vi "find object distance in direction.vi"(9 "direction":dbl, 10 "point":cluster{"x":i16, "y":i16}, 11 "raster image":bool[][](array[boolean])) -> (2 "distance":sgl)   [LabVIEW 2009]
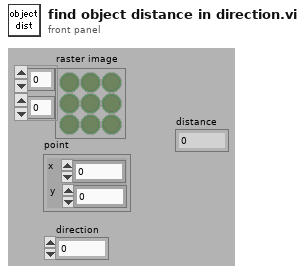
[diagram p1: front panel]
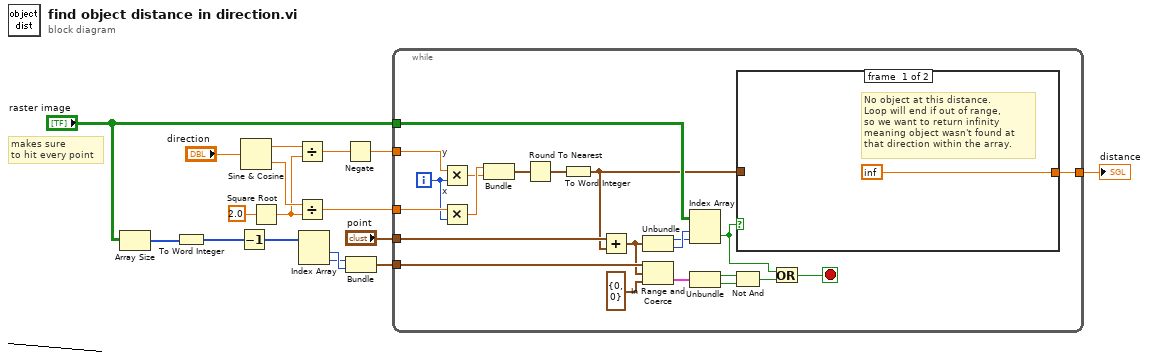
[diagram p0: block diagram]
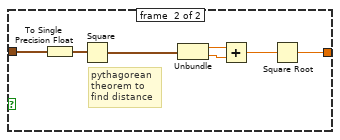
[diagram p2: hidden frame]
diagram:
  # "makes sure\nto hit every point"
  n1 = Array Size(array="raster image") -> (size(s)=w7:i32[])
  n2 = To Word Integer(number=w7) -> (16bit integer=w5:i16[])
  n3 = Decrement(x=w5) -> (x-1=w6:i16[])
  n4 = Sine & Cosine(0:"direction") -> (1:w14:dbl, 2:w15:dbl)
  n5 = Square Root(x=2.0) -> (sqrt(x)=w13:dbl)
  n6 = Divide(x=w14, y=w13) -> (x/y=w12:dbl)
  n7 = Divide(x=w15, y=w13) -> (x/y=w11:dbl)
  n8 = Index Array(array=w6) -> (element #1=w3:i16, element #2=w2:i16)  [unwired: 2 in]
  n9 = Negate(x=w12) -> (-x=w10:dbl)
  n10 = Bundle(w2, w3) -> (w4:cluster{i16, i16})  [unwired: 1 in]
  n11 = while {
    tunnel: w10 -> [w37]
    tunnel: w11 -> [w39]
    tunnel: "point" -> [w32]
    tunnel: "raster image" -> [w29]
    tunnel: w4 -> [w31]
    tunnel: [w23] -> w1
    i -> [w38]
    stop <- w25 stop-if-true
    n12 = Multiply "y"(x=w37, y=w38) -> (x*y=w35:dbl)
    n13 = Multiply "x"(x=w39, y=w38) -> (x*y=w36:dbl)
    n14 = Bundle(w36, w35) -> (w34:cluster{dbl, dbl})  [unwired: 1 in]
    n15 = Round To Nearest(number=w34) -> (nearest integer value=w33:cluster{dbl, dbl})
    n16 = To Word Integer(number=w33) -> (16bit integer=w24:cluster{i16, i16})
    n17 = Add(x=w32, y=w24) -> (x+y=w26:cluster{i16, i16})
    n18 = Unbundle(w26) -> (w27:i16, w28:i16)
    n19 = In Range and Coerce(upper limit=w31, x=w26, lower limit=cluster{i16, i16} {0, 0}) -> (In Range?=w22:cluster{bool, bool})  [unwired: 1 out]
    n20 = Index Array(array=w29, index (row)=w28, index (col)=w27) -> (element=w21:bool)
    n21 = Unbundle(w22) -> (w20:bool, w19:bool)
    n22 = Not And(1:w19, 2:w20) -> (0:w18:bool)
    n23 = case shown="False" w21 {
      tunnel: w24 -> [_ w47]
      tunnel: [sgl inf w41] -> w23
      frame #0 {
        # "No object at this distance.\nLoop will end if out of range,\nso we want to return infinity\nmeaning object wasn't found at \nthat direction within the array."
      }
      frame #1 {
        # "pythagorean\ntheorem to\nfind distance"
        n24 = To Single Precision Float(number=w47) -> (single precision float=w43:cluster{sgl, sgl})
        n25 = Square(x=w43) -> (x^2=w46:cluster{sgl, sgl})
        n26 = Unbundle(w46) -> (w45:sgl, w44:sgl)
        n27 = Add(x=w45, y=w44) -> (x+y=w42:sgl)
        n28 = Square Root(x=w42) -> (sqrt(x)=w41:sgl)
      }
    }
    n29 = Or(x=w21, y=w18) -> (x .or. y?=w25:bool)
  }
  "distance" <- w1
